vi "matgen.vi"(8 "v4":dbl, 9 "v3":dbl, 10 "v2":dbl, 11 "v1":dbl) -> (3 "B":dbl[][](array[numeric]))   [LabVIEW 2015]
uses:
  <vilib>/imath/engines/lvmath2/RunTimeEngine/NodeEndStatement/NIMS_NodeEndStatement_Output.vi
  <instcachedir>/0/NIMS_NodeEndStatement_Output_53EC0D466D134D7ABD903AC30B43404B.lvgen/NIMS_NodeEndStatement_Output_53EC0D466D134D7ABD903AC30B43404B_002.vi
  <vilib>/imath/engines/lvmath2/RunTimeEngine/ErrorHandling/NIMS_Finalize Error.vi
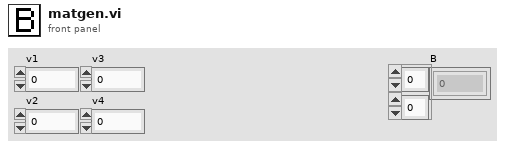
[diagram p1: front panel]
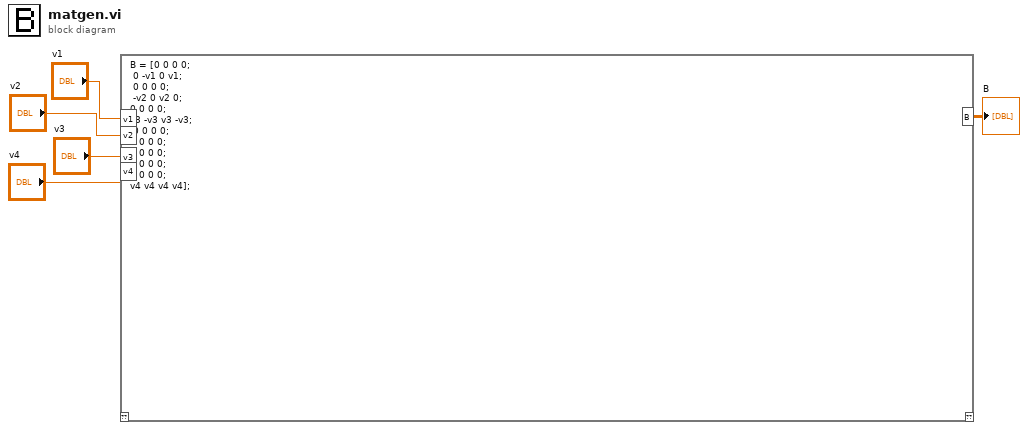
[diagram p0: block diagram]
diagram:
  n1 = mathscript code="B = [0 0 0 0;\n 0 -v1 0 v1;\n 0 0 0 0;\n -v2 0 v2 0;\n0 0 0 0;\nv3 -v3 v3 -v3;\n 0 0 0 0;\n0 0 0 0;\n0 0 0 0;\n0 0 0 0;\n0 0 0 0;\nv4 v4 v4 v4];"("v1"="v1", "v2"="v2", "v3"="v3", "v4"="v4") -> ("B"=→"B":dbl[][])  [unwired: 1 in, 1 out]
